vi "Gestore prove.vi"(8 "banco":i32, 9 "Status":refnum<vi>, 11 "Queue Name":string) -> ()   [LabVIEW 2019]
uses:
  TypeDef/Cluster INFO.ctl
  TypeDef/WT SELECTION.ctl
  TypeDef/Definizione linea.ctl
  TypeDef/Collegamenti_elettrici.ctl
  TypeDef/Control Calcoli.ctl
  Global prova in corso.vi
panel:
  out "Scale misura res":T1
  out "%VALVOLE":dbl[][](array[numeric])
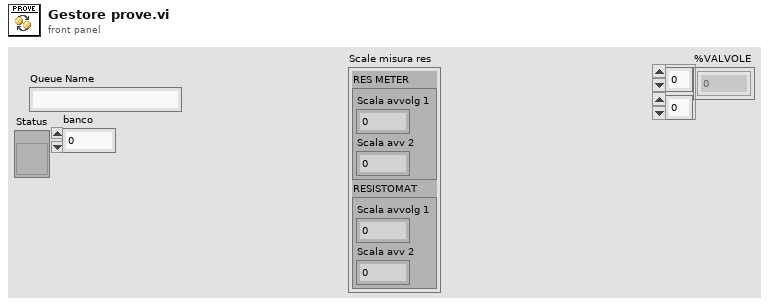
[diagram p1: front panel]
types:
  T1 = cluster{"RES METER":cluster{"Scala avvolg 1":u16, "Scala avv 2":u16}, "RESISTOMAT":cluster{"Scala avvolg 1":u16, "Scala avv 2":u16}}
  T2 = typedef "Cluster INFO.ctl" = cluster{"Scelta wattmetro":cluster{"Wattmetro":T3}, "SET RPM":dbl, "SET TEMP":dbl, "Array banchi":T4[], "Array valvole linee avvio/fermata":cluster{"Valvole avvio":cluster{"Set valvole avvio?":bool, "% valvole avvio":dbl[]}, "Valvole fermata":cluster{"Set valvole fermata?":bool, "% valvole fermata":dbl[]}}[], "banco selezionato":i8, "Nomi valvole prop sistema":string[], "canale-- sensore":string[][], "Attriti B1":dbl[][], "Attriti B2":dbl[][], "Collegamento elettrico":cluster{"ALIMENTAZIONE ELETTRICA":T5, "ID":i16, "#rami freddo\\eq term resmeter":i16, "#rami riscaldamento resmeter":i16, "#rami freddo\\eq term resistomat":i16, "#rami riscaldamento resistomat":i16, "CALCOLI":T6}, "lingua":i16, "Costanti collaudo":cluster{"P [bar]":dbl, "T amb. [°C]":dbl, "Umidità [%]":dbl, "T acqua [°C] 2":dbl}, "OPZIONI MISURE RES":cluster{"MISURA A FREDDO":enum16{"NESSUNO", "RESISTOMAT", "RES METER", "ENTRAMBI"}, "MISURA EQ. TERMICO":enum16{"NESSUNO", "RESISTOMAT", "RES METER", "ENTRAMBI"}, "MISURA DT PROVA IN CORSO":enum16{"NESSUNO", "RESISTOMAT - CON FERMATE", "RES METER - CON FERMATE", "RES METER - CONTINUO"}, "MISURE PRIMA E DOPO":enum16{"NESSUNO", "RESISTOMAT", "RES METER"}, "STRUMENTI PRESENTI":enum16{"NESSUNO", "RESISTOMAT", "RES METER", "ENTRAMBI"}}, "Dati targa motore":cluster{"Vnom":dbl, "Fnom":dbl, "Inom":dbl, "Cnom":dbl, "Npoli":dbl, "Scorta 1":dbl, "Scorta 2":dbl, "Scorta 3":dbl}}
  T3 = typedef "WT SELECTION.ctl" = enum32{"No Selection", "WT230", "WT1600", "WT1800", "WT330", "VIW", "APLUS"}
  T4 = typedef "Definizione linea.ctl" = cluster{"Nome":string, "Tors. scala1":i32, "Tors. scala2":i32, "rpm":i32, "TAMB":i32, "Indici Temperature":i16[], "Indice freno":i16, "alimentatore trifase":i16, "alimentatore monofase":i16, "alimentatore dc arm":i16, "alimentatore dc ecc":i16, "alimentatore dc mp":i16}
  T5 = typedef "Collegamenti_elettrici.ctl" = enum16{"AC TRIFASE", "AC TRIFASE + FRENO", "AC MONOFASE", "DC CON ECCITAZIONE", "DC CON ECCITAZIONE + FRENO", "DC NO ECCITAZIONE", "DC NO ECCITAZIONE + FRENO", "FRENO TRASC + AFE", "SOLO FRENO", "CARICO RESISTIVO", "GENERICO", "SOLO ACQUISITORE", "SCORTA 4", "SCORTA 5", "SCORTA 6"}
  T6 = typedef "Control Calcoli.ctl" = enum16{"AC TRIFASE", "AC MONOFASE", "DC ECCITAZIONE", "DC NO ECCITAZIONE", "POMPA TRIFASE", "POMPA MONOFASE", "GENERICO", "TRASFORMATORE", "ALTERNATORE TRASCINATO", "GRUPPO ELETTROGENO"}
  T7 = cluster{"Array of elements":cluster{"String":string, "variant":variant}[], "Single element":cluster{"String":string, "variant":variant}, "enque at\nopposite end (F)":bool, "no replications (F)":bool}
  T8 = cluster{"Prova":string, "MAN/AUTO":bool, "Tipo motore pompa":enum16{"Monofase", "Trifase"}}
  T9 = cluster{"Res Ch1":dbl, "Res Ch2":dbl, "tAMB":dbl, "Res Ch3":dbl}
  T10 = cluster{"Res Ch1":dbl, "Res Ch2":dbl, "tAMB":dbl}
  T11 = cluster{"ALIMENTAZIONE ELETTRICA":T5, "ID":i16, "#rami freddo\\eq term resmeter":i16, "#rami riscaldamento resmeter":i16, "#rami freddo\\eq term resistomat":i16, "#rami riscaldamento resistomat":i16, "CALCOLI":T6}
  T12 = cluster{"MISURA A FREDDO":enum16{"NESSUNO", "RESISTOMAT", "RES METER", "ENTRAMBI"}, "MISURA EQ. TERMICO":enum16{"NESSUNO", "RESISTOMAT", "RES METER", "ENTRAMBI"}, "MISURA DT PROVA IN CORSO":enum16{"NESSUNO", "RESISTOMAT - CON FERMATE", "RES METER - CON FERMATE", "RES METER - CONTINUO"}, "MISURE PRIMA E DOPO":enum16{"NESSUNO", "RESISTOMAT", "RES METER"}, "STRUMENTI PRESENTI":enum16{"NESSUNO", "RESISTOMAT", "RES METER", "ENTRAMBI"}}
  T13 = enum16{"NESSUNO", "RESISTOMAT", "RES METER", "ENTRAMBI"}
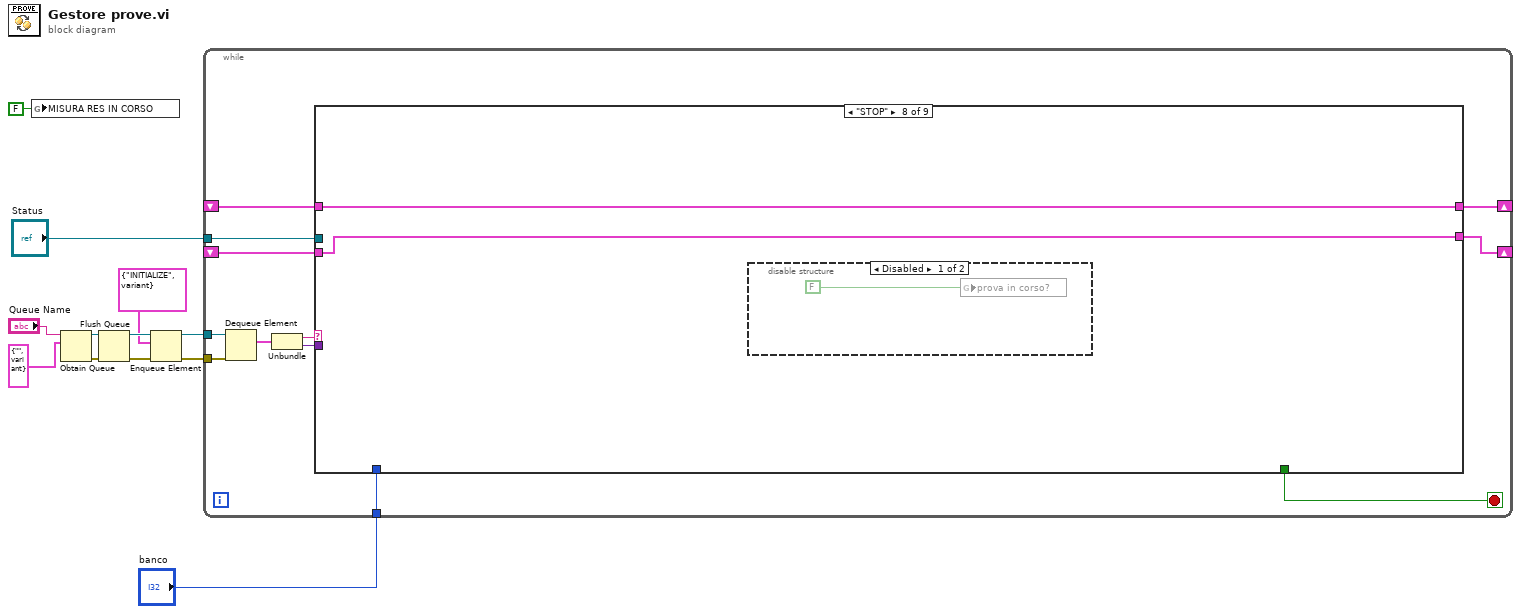
[diagram p0: block diagram]
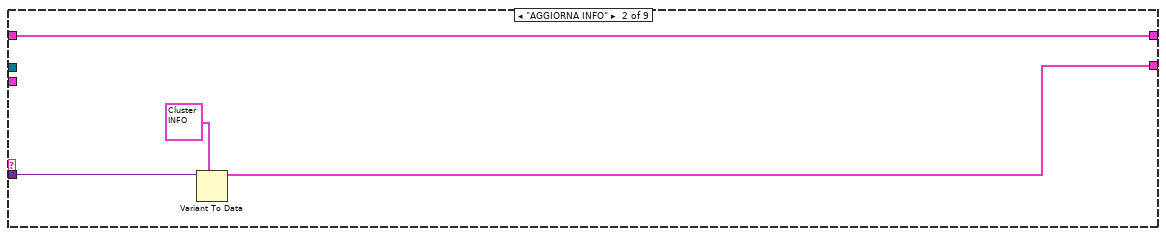
[diagram p3: hidden frame]
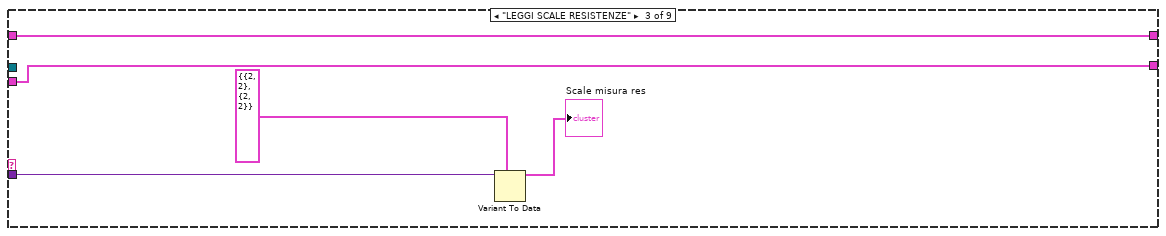
[diagram p4: hidden frame]
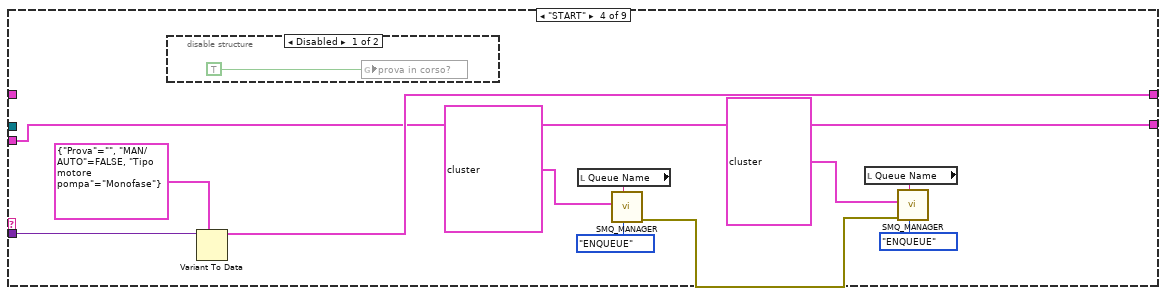
[diagram p5: hidden frame]
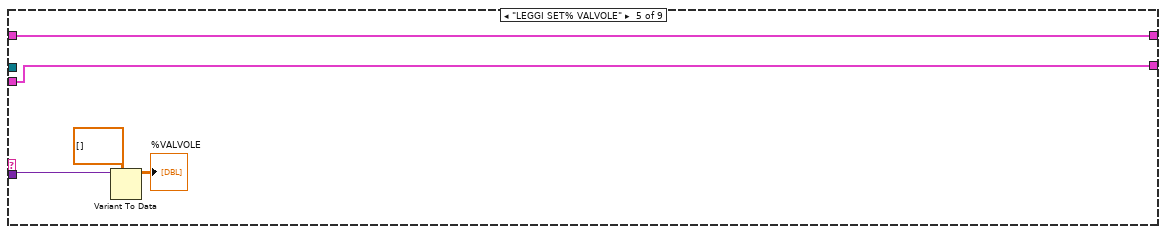
[diagram p7: hidden frame]
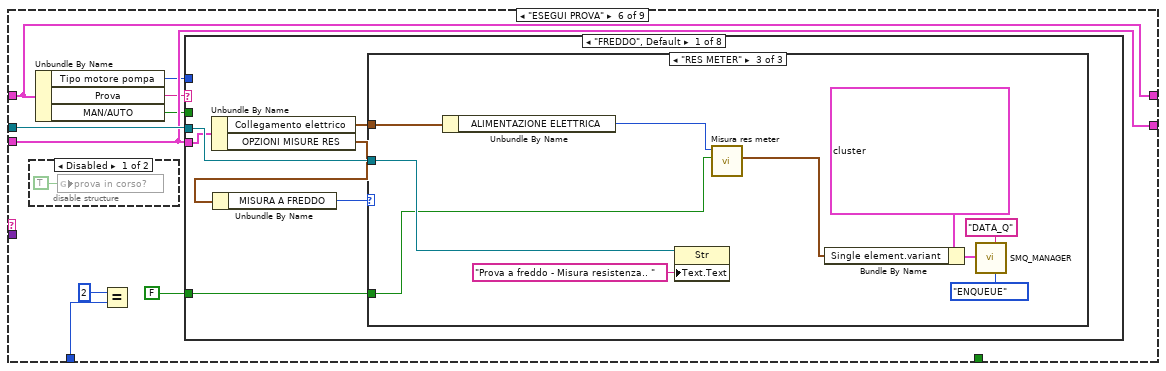
[diagram p8: hidden frame]
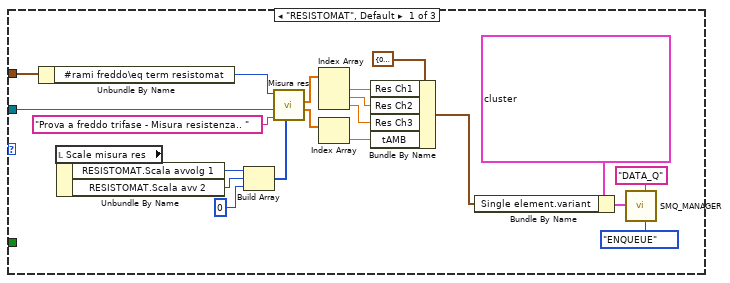
[diagram p10: hidden frame]
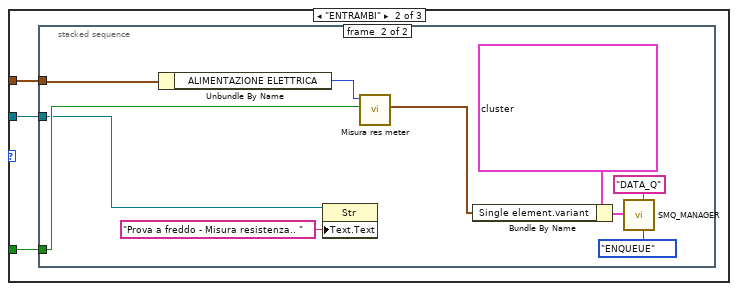
[diagram p11: hidden frame]
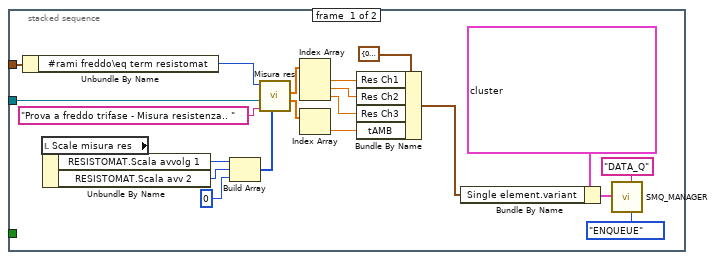
[diagram p12: hidden frame]
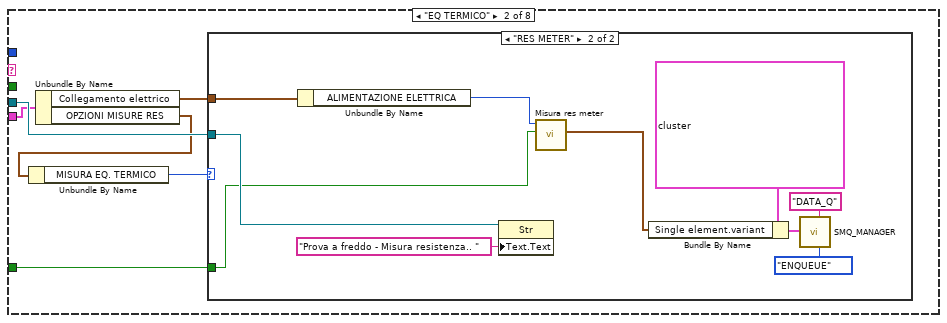
[diagram p13: hidden frame]
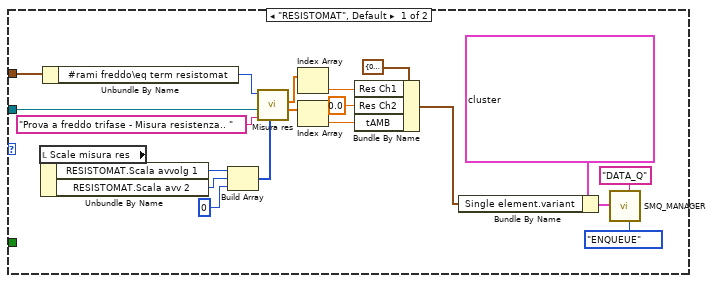
[diagram p14: hidden frame]
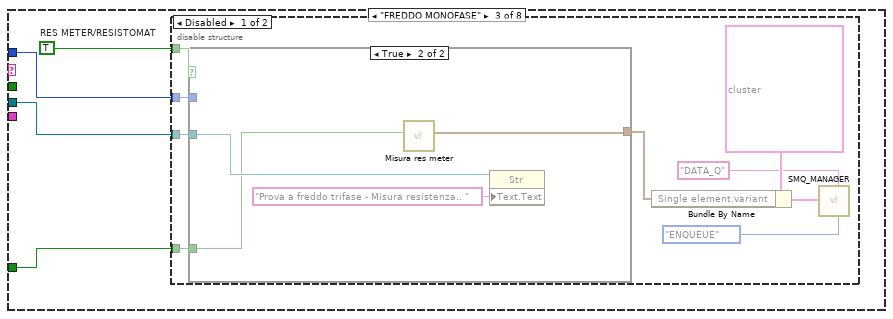
[diagram p15: hidden frame]
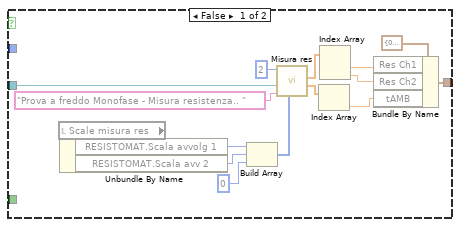
[diagram p16: hidden frame]
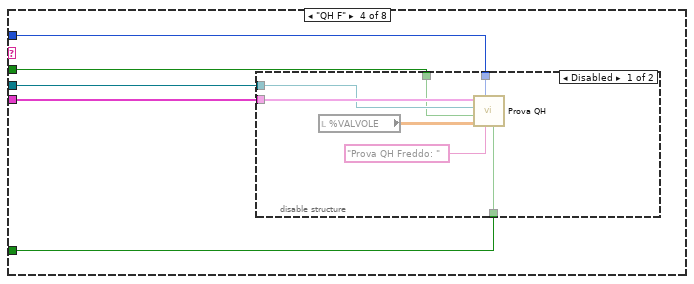
[diagram p18: hidden frame]
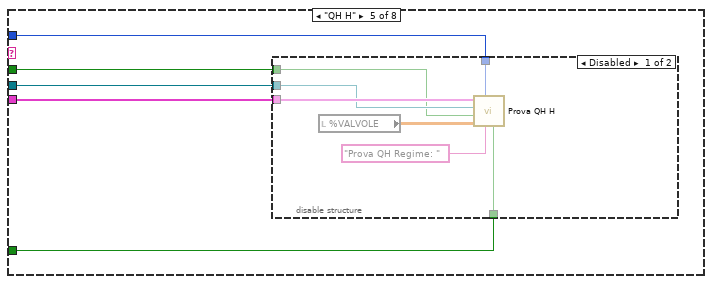
[diagram p20: hidden frame]
diagram:
  n1 = global write "Global prova in corso.vi" "MISURA RES IN CORSO"(FALSE ("prova in corso?")) -> ()
  n2 = Obtain Queue(name (unnamed)="Queue Name", element data type=cluster{"String":string, "variant":variant} {"String"="", "variant"=variant} ("element")) -> (queue out=w6:refnum<queue>, error out=w7:errorcluster)  [unwired: 3 in, 1 out]
  n3 = Flush Queue(queue=w6, error in (no error)=w7) -> (queue out=w9:refnum<queue>, error out=w10:errorcluster)  [unwired: 1 out]
  n4 = Enqueue Element(queue=w9, element=cluster{"String":string, "variant":variant} {"String"="INITIALIZE", "variant"=variant}, error in (no error)=w10) -> (queue out=w11:refnum<queue>, error out=w12:errorcluster)  [unwired: 1 in, 1 out]
  n5 = while {
    tunnel: w11 -> [w23]
    tunnel: w12 -> [w22]
    shift-right: [w19] -> _
    shift-left: _ -> [w18]
    tunnel: "Status" -> [w17]
    shift-right: [w15] -> _
    shift-left: _ -> [w14]
    tunnel: "banco" -> [w13]
    stop <- w16 stop-if-true
    n6 = Dequeue Element(queue=w23, error in (no error)=w22) -> (element=w24:cluster{"String":string, "variant":variant})  [unwired: 1 in, 3 out]
    n7 = Unbundle(w24) -> ("String"=w21:string, "variant"=w20:variant)
    n8 = case shown="\"STOP\"" w21 {
      tunnel: w20 -> [_ w30 w35 w43 w50 _ _ _ _]
      tunnel: [w26 w29 w33 w42 w52 w59 w261 w263 w266] -> w19
      tunnel: w18 -> [w26 w29 w33 _ w52 w59 w261 w263 w266]
      tunnel: w17 -> [_ _ _ _ _ w61 _ _ _]
      tunnel: [_ _ _ _ _ _ _ _ TRUE] -> w16
      tunnel: [w25 w28 w32 w41 w51 w60 w260 w262 w265] -> w15
      tunnel: w14 -> [w25 _ w32 w41 w51 w60 w260 w262 w265]
      tunnel: w13 -> [_ _ _ _ _ w55 _ _ _]
      frame "INITIALIZE", Default {
      }
      frame "AGGIORNA INFO" {
        n9 = Variant To Data(type=T2 {"Scelta wattmetro"={"Wattmetro"=enum."No Selection"}, "SET RPM"=0.0, "SET TEMP"=0.0, "Array banchi"=[{"Nome"="Elettropompa", "Tors. scala1"=0, "Tors. scala2"=0, "rpm"=0, "TAMB"=0, "Indici Temperature"=[0, 1], "Indice freno"=1, "alimentatore trifase"=0, "alimentatore monofase"=0, "alimentatore dc arm"=0, "alimentatore dc ecc"=0, "alimentatore dc mp"=0}, {"Nome"="Sommersa", "Tors. scala1"=0, "Tors. scala2"=0, "rpm"=0, "TAMB"=1, "Indici Temperature"=[0, 1], "Indice freno"=0, "alimentatore trifase"=0, "alimentatore monofase"=0, "alimentatore dc arm"=0, "alimentatore dc ecc"=0, "alimentatore dc mp"=0}], "Array valvole linee avvio/fermata"=[], "banco selezionato"=0, "Nomi valvole prop sistema"=[], "canale-- sensore"=[], "Attriti B1"=[], "Attriti B2"=[], "Collegamento elettrico"={"ALIMENTAZIONE ELETTRICA"=enum."AC TRIFASE", "ID"=0, "#rami freddo\\eq term resmeter"=0, "#rami riscaldamento resmeter"=0, "#rami freddo\\eq term resistomat"=0, "#rami riscaldamento resistomat"=0, "CALCOLI"=enum."AC TRIFASE"}, "lingua"=0, "Costanti collaudo"={"P [bar]"=0.0, "T amb. [°C]"=0.0, "Umidità [%]"=0.0, "T acqua [°C] 2"=0.0}, "OPZIONI MISURE RES"={"MISURA A FREDDO"=enum."RESISTOMAT", "MISURA EQ. TERMICO"=enum."RESISTOMAT", "MISURA DT PROVA IN CORSO"=enum."RESISTOMAT - CON FERMATE", "MISURE PRIMA E DOPO"=enum."RESISTOMAT", "STRUMENTI PRESENTI"=enum."NESSUNO"}, "Dati targa motore"={"Vnom"=0.0, "Fnom"=0.0, "Inom"=0.0, "Cnom"=0.0, "Npoli"=0.0, "Scorta 1"=0.0, "Scorta 2"=0.0, "Scorta 3"=0.0}} ("Cluster INFO"), Variant=w30) -> (data=w28:T2)  [unwired: 1 in, 1 out]
      }
      frame "LEGGI SCALE RESISTENZE" {
        n10 = Variant To Data(type=T1 {"RES METER"={"Scala avvolg 1"=2, "Scala avv 2"=2}, "RESISTOMAT"={"Scala avvolg 1"=2, "Scala avv 2"=2}} ("Scale Misura res"), Variant=w35) -> (data=→"Scale misura res":T1)  [unwired: 1 in, 1 out]
      }
      frame "START" {
        n11 = disable-structure shown="Disabled" {
          frame Disabled {
            n12 = global write "Global prova in corso.vi" "prova in corso?"(TRUE ("prova in corso?")) -> ()
          }
          frame Enabled {
          }
        }
        n13 = Variant To Data(type=T8 {"Prova"="", "MAN/AUTO"=FALSE, "Tipo motore pompa"=enum."Monofase"} ("output cluster"), Variant=w43) -> (data=w42:T8)  [unwired: 1 in, 1 out]
        n14 = local read "Queue Name"() -> (w45:string)
        n15 = call <userlib>:"SMQ_MANAGER.vi"("Function"=enum16{"INITIALIZE", "ENQUEUE", "STOP ALL"}."ENQUEUE", "Queue name"=w45, "Enqueue cluster"=T7 {"Array of elements"=[], "Single element"={"String"="ESEGUI PROVA", "variant"=variant}, "enque at\nopposite end (F)"=FALSE, "no replications (F)"=FALSE}) -> ("error out"=w36:errorcluster)  [unwired: 8 in]
        n16 = local read "Queue Name"() -> (w38:string)
        n17 = call <userlib>:"SMQ_MANAGER.vi"("Function"=enum16{"INITIALIZE", "ENQUEUE", "STOP ALL"}."ENQUEUE", "Queue name"=w38, "error in (no error)"=w36, "Enqueue cluster"=T7 {"Array of elements"=[], "Single element"={"String"="FINE PROVA", "variant"=variant}, "enque at\nopposite end (F)"=FALSE, "no replications (F)"=FALSE}) -> ()  [unwired: 7 in, 1 out]
      }
      frame "LEGGI SET% VALVOLE" {
        n18 = Variant To Data(type=dbl[][] [], Variant=w50) -> (data=→"%VALVOLE":dbl[][])  [unwired: 1 in, 1 out]
      }
      frame "ESEGUI PROVA" {
        n19 = disable-structure shown="Disabled" {
          frame Disabled {
            n20 = global write "Global prova in corso.vi" "prova in corso?"(TRUE ("prova in corso?")) -> ()
          }
          frame Enabled {
          }
        }
        n21 = Unbundle By Name(w59) -> ("Tipo motore pompa"=w57:enum16{"Monofase", "Trifase"}, "Prova"=w58:string, "MAN/AUTO"=w56:bool)
        n22 = Equal?(x=2, y=w55) -> ()  [unwired: 1 out]
        n23 = case shown="\"FREDDO\", Default" w58 {
          tunnel: w61 -> [w68 w139 w173 w205 w217 w228 w237 w251]
          tunnel: w60 -> [w66 w137 _ w206 w218 w229 w239 w253]
          tunnel: w57 -> [_ _ w170 w204 w216 w227 w238 w252]
          tunnel: w56 -> [_ _ _ w203 w215 _ _ w250]
          tunnel: FALSE -> [w67 w138 w171 w202 w214 w226 w236 _]
          frame "FREDDO", Default {
            n24 = Unbundle By Name(w66) -> ("Collegamento elettrico"=w63:T11, "OPZIONI MISURE RES"=w65:T12)
            n25 = Unbundle By Name(w65) -> ("MISURA A FREDDO"=w64:T13)
            n26 = case shown="\"RES METER\"" w64 {
              tunnel: w68 -> [w89 w92 w133]
              tunnel: w67 -> [_ w90 w131]
              tunnel: w63 -> [w74 w91 w125]
              frame "RESISTOMAT", Default {
                n27 = Unbundle By Name(w74) -> ("#rami freddo\\eq term resistomat"=w73:i16)
                n28 = local read "Scale misura res"() -> (w88:T1)
                n29 = Unbundle By Name(w88) -> ("RESISTOMAT.Scala avvolg 1"=w87:u16, "RESISTOMAT.Scala avv 2"=w86:u16)
                n30 = Build Array(w87, w86, u16 0 ("element")) -> (w85:u16[])
                n31 = call "Misura res.vi"("Scala per ramo"=w85, "String"="Prova a freddo trifase - Misura resistenza.. ", "Status"=w89, "N°rami"=w73) -> ("temperature amb"=w82:dbl[], "Valori res (ohm)"=w81:dbl[])  [unwired: 5 in, 1 out]
                n32 = Index Array(array=w81) -> (element #1=w80:dbl, element #2=w70:dbl, element #3=w69:dbl)  [unwired: 3 in]
                n33 = Index Array(array=w82) -> (element=w71:dbl)  [unwired: 1 in]
                n34 = Bundle By Name(cluster=T9 {"Res Ch1"=0.0, "Res Ch2"=0.0, "tAMB"=0.0, "Res Ch3"=0.0} ("FREDDO resistomat"), "Res Ch1"=w80, "Res Ch2"=w70, "Res Ch3"=w69, "tAMB"=w71) -> (w75:T9)
                n35 = Bundle By Name(cluster=T7 {"Array of elements"=[], "Single element"={"String"="READ RES FREDDO RESISTOMAT", "variant"=variant}, "enque at\nopposite end (F)"=FALSE, "no replications (F)"=FALSE} ("Enqueue cluster"), "Single element.variant"=w75) -> (w79:T7)
                n36 = call <userlib>:"SMQ_MANAGER.vi"("Function"=enum16{"INITIALIZE", "ENQUEUE", "STOP ALL"}."ENQUEUE", "Queue name"="DATA_Q", "Enqueue cluster"=w79) -> ()  [unwired: 8 in, 1 out]
              }
              frame "ENTRAMBI" {
                n37 = stacked-sequence {
                  tunnel: w92 -> [w113 w114]
                  tunnel: w91 -> [w98 w116]
                  tunnel: w90 -> [_ w115]
                  frame #0 {
                    n38 = Unbundle By Name(w98) -> ("#rami freddo\\eq term resistomat"=w97:i16)
                    n39 = local read "Scale misura res"() -> (w112:T1)
                    n40 = Unbundle By Name(w112) -> ("RESISTOMAT.Scala avvolg 1"=w111:u16, "RESISTOMAT.Scala avv 2"=w110:u16)
                    n41 = Build Array(w111, w110, u16 0 ("element")) -> (w109:u16[])
                    n42 = call "Misura res.vi"("Scala per ramo"=w109, "String"="Prova a freddo trifase - Misura resistenza.. ", "Status"=w113, "N°rami"=w97) -> ("temperature amb"=w106:dbl[], "Valori res (ohm)"=w105:dbl[])  [unwired: 5 in, 1 out]
                    n43 = Index Array(array=w105) -> (element #1=w104:dbl, element #2=w94:dbl, element #3=w93:dbl)  [unwired: 3 in]
                    n44 = Index Array(array=w106) -> (element=w95:dbl)  [unwired: 1 in]
                    n45 = Bundle By Name(cluster=T9 {"Res Ch1"=0.0, "Res Ch2"=0.0, "tAMB"=0.0, "Res Ch3"=0.0} ("FREDDO resistomat"), "Res Ch1"=w104, "Res Ch2"=w94, "Res Ch3"=w93, "tAMB"=w95) -> (w99:T9)
                    n46 = Bundle By Name(cluster=T7 {"Array of elements"=[], "Single element"={"String"="READ RES FREDDO RESISTOMAT", "variant"=variant}, "enque at\nopposite end (F)"=FALSE, "no replications (F)"=FALSE} ("Enqueue cluster"), "Single element.variant"=w99) -> (w103:T7)
                    n47 = call <userlib>:"SMQ_MANAGER.vi"("Function"=enum16{"INITIALIZE", "ENQUEUE", "STOP ALL"}."ENQUEUE", "Queue name"="DATA_Q", "Enqueue cluster"=w103) -> ()  [unwired: 8 in, 1 out]
                  }
                  frame #1 {
                    n48 = Unbundle By Name(w116) -> ("ALIMENTAZIONE ELETTRICA"=w117:T5)
                    n49 = property class="Str"(reference=w114, "Text.Text"="Prova a freddo - Misura resistenza.. " ("String")) -> ()  [unwired: 1 in, 2 out]
                    n50 = call "Misura res meter.vi"("solo lettura?"=w115, "ALIMENTAZIONE ELETTRICA"=w117) -> ("FREDDO"=w118:T9)  [unwired: 9 in]
                    n51 = Bundle By Name(cluster=T7 {"Array of elements"=[], "Single element"={"String"="READ RES FREDDO RES METER", "variant"=variant}, "enque at\nopposite end (F)"=FALSE, "no replications (F)"=FALSE} ("Enqueue cluster"), "Single element.variant"=w118) -> (w122:T7)
                    n52 = call <userlib>:"SMQ_MANAGER.vi"("Function"=enum16{"INITIALIZE", "ENQUEUE", "STOP ALL"}."ENQUEUE", "Queue name"="DATA_Q", "Enqueue cluster"=w122) -> ()  [unwired: 8 in, 1 out]
                  }
                }
              }
              frame "RES METER" {
                n53 = Unbundle By Name(w125) -> ("ALIMENTAZIONE ELETTRICA"=w124:T5)
                n54 = property class="Str"(reference=w133, "Text.Text"="Prova a freddo - Misura resistenza.. " ("String")) -> ()  [unwired: 1 in, 2 out]
                n55 = call "Misura res meter.vi"("solo lettura?"=w131, "ALIMENTAZIONE ELETTRICA"=w124) -> ("FREDDO"=w126:T9)  [unwired: 9 in]
                n56 = Bundle By Name(cluster=T7 {"Array of elements"=[], "Single element"={"String"="READ RES FREDDO RES METER", "variant"=variant}, "enque at\nopposite end (F)"=FALSE, "no replications (F)"=FALSE} ("Enqueue cluster"), "Single element.variant"=w126) -> (w130:T7)
                n57 = call <userlib>:"SMQ_MANAGER.vi"("Function"=enum16{"INITIALIZE", "ENQUEUE", "STOP ALL"}."ENQUEUE", "Queue name"="DATA_Q", "Enqueue cluster"=w130) -> ()  [unwired: 8 in, 1 out]
              }
            }
          }
          frame "EQ TERMICO" {
            n58 = Unbundle By Name(w137) -> ("Collegamento elettrico"=w134:T11, "OPZIONI MISURE RES"=w136:T12)
            n59 = Unbundle By Name(w136) -> ("MISURA EQ. TERMICO"=w135:T13)
            n60 = case shown="\"RES METER\"" w135 {
              tunnel: w139 -> [w159 w169]
              tunnel: w138 -> [_ w167]
              tunnel: w134 -> [w141 w161]
              frame "RESISTOMAT", Default {
                n61 = local read "Scale misura res"() -> (w158:T1)
                n62 = Unbundle By Name(w158) -> ("RESISTOMAT.Scala avvolg 1"=w157:u16, "RESISTOMAT.Scala avv 2"=w156:u16)
                n63 = Unbundle By Name(w141) -> ("#rami freddo\\eq term resistomat"=w140:i16)
                n64 = Build Array(w157, w156, u16 0 ("element")) -> (w155:u16[])
                n65 = call "Misura res.vi"("Scala per ramo"=w155, "String"="Prova a freddo trifase - Misura resistenza.. ", "Status"=w159, "N°rami"=w140) -> ("temperature amb"=w152:dbl[], "Valori res (ohm)"=w148:dbl[])  [unwired: 5 in, 1 out]
                n66 = Index Array(array=w148) -> (element=w147:dbl)  [unwired: 1 in]
                n67 = Index Array(array=w152) -> (element=w150:dbl)  [unwired: 1 in]
                n68 = Bundle By Name(cluster=T10 {"Res Ch1"=0.0, "Res Ch2"=0.0, "tAMB"=0.0} ("Cluster FREDDO"), "Res Ch1"=w147, "Res Ch2"=0.0, "tAMB"=w150) -> (w142:T10)
                n69 = Bundle By Name(cluster=T7 {"Array of elements"=[], "Single element"={"String"="READ RES FREDDO RESISTOMAT", "variant"=variant}, "enque at\nopposite end (F)"=FALSE, "no replications (F)"=FALSE} ("Enqueue cluster"), "Single element.variant"=w142) -> (w146:T7)
                n70 = call <userlib>:"SMQ_MANAGER.vi"("Function"=enum16{"INITIALIZE", "ENQUEUE", "STOP ALL"}."ENQUEUE", "Queue name"="DATA_Q", "Enqueue cluster"=w146) -> ()  [unwired: 8 in, 1 out]
              }
              frame "RES METER" {
                n71 = Unbundle By Name(w161) -> ("ALIMENTAZIONE ELETTRICA"=w160:T5)
                n72 = property class="Str"(reference=w169, "Text.Text"="Prova a freddo - Misura resistenza.. " ("String")) -> ()  [unwired: 1 in, 2 out]
                n73 = call "Misura res meter.vi"("solo lettura?"=w167, "ALIMENTAZIONE ELETTRICA"=w160) -> ("FREDDO"=w162:T9)  [unwired: 9 in]
                n74 = Bundle By Name(cluster=T7 {"Array of elements"=[], "Single element"={"String"="READ RES FREDDO RESISTOMAT", "variant"=variant}, "enque at\nopposite end (F)"=FALSE, "no replications (F)"=FALSE} ("Enqueue cluster"), "Single element.variant"=w162) -> (w166:T7)
                n75 = call <userlib>:"SMQ_MANAGER.vi"("Function"=enum16{"INITIALIZE", "ENQUEUE", "STOP ALL"}."ENQUEUE", "Queue name"="DATA_Q", "Enqueue cluster"=w166) -> ()  [unwired: 8 in, 1 out]
              }
            }
          }
          frame "FREDDO MONOFASE" {
            w172 = TRUE  # RES METER/RESISTOMAT
            n76 = disable-structure shown="Disabled" {
              disable-tunnel: w173 -> [w182 _]
              disable-tunnel: w172 -> [w176 _]
              disable-tunnel: w171 -> [w175 _]
              disable-tunnel: w170 -> [w174 _]
              frame Disabled {
                n77 = case shown="True" w176 {
                  tunnel: w182 -> [w197 w200]
                  tunnel: [w186 w201] -> w177
                  tunnel: w175 -> [_ w198]
                  tunnel: w174 -> [_ _]
                  frame False {
                    n78 = local read "Scale misura res"() -> (w196:T1)
                    n79 = Unbundle By Name(w196) -> ("RESISTOMAT.Scala avvolg 1"=w195:u16, "RESISTOMAT.Scala avv 2"=w194:u16)
                    n80 = Build Array(w195, w194, u16 0 ("element")) -> (w193:u16[])
                    n81 = call "Misura res.vi"("Scala per ramo"=w193, "String"="Prova a freddo Monofase - Misura resistenza.. ", "Status"=w197, "N°rami"=2) -> ("temperature amb"=w189:dbl[], "Valori res (ohm)"=w185:dbl[])  [unwired: 5 in, 1 out]
                    n82 = Index Array(array=w189) -> (element=w187:dbl)  [unwired: 1 in]
                    n83 = Index Array(array=w185) -> (element #1=w184:dbl, element #2=w183:dbl)  [unwired: 2 in]
                    n84 = Bundle By Name(cluster=T10 {"Res Ch1"=0.0, "Res Ch2"=0.0, "tAMB"=0.0} ("Cluster FREDDO"), "Res Ch1"=w184, "Res Ch2"=w183, "tAMB"=w187) -> (w186:T10)
                  }
                  frame True {
                    n85 = call "Misura res meter.vi"("solo lettura?"=w198) -> ("FREDDO"=w201:T9)  [unwired: 10 in]
                    n86 = property class="Str"(reference=w200, "Text.Text"="Prova a freddo trifase - Misura resistenza.. " ("String")) -> ()  [unwired: 1 in, 2 out]
                  }
                }
                n87 = Bundle By Name(cluster=T7 {"Array of elements"=[], "Single element"={"String"="READ RES FREDDO", "variant"=variant}, "enque at\nopposite end (F)"=FALSE, "no replications (F)"=FALSE} ("Enqueue cluster"), "Single element.variant"=w177) -> (w181:T7)
                n88 = call <userlib>:"SMQ_MANAGER.vi"("Function"=enum16{"INITIALIZE", "ENQUEUE", "STOP ALL"}."ENQUEUE", "Queue name"="DATA_Q", "Enqueue cluster"=w181) -> ()  [unwired: 8 in, 1 out]
              }
              frame Enabled {
              }
            }
          }
          frame "QH F" {
            n89 = disable-structure shown="Disabled" {
              disable-tunnel: w206 -> [w213 _]
              disable-tunnel: w205 -> [w212 _]
              disable-tunnel: w204 -> [w211 _]
              disable-tunnel: w203 -> [w210 _]
              disable-tunnel: w202 -> [w207 _]
              frame Disabled {
                n90 = local read "%VALVOLE"() -> (w209:dbl[][])
                n91 = call "Prova QH.vi"("solo acquisizione!!"=w207, "Text.Text"="Prova QH Freddo: ", "Tipo motore pompa"=w211, "Array % valvole"=w209, "Manuale F\\auto T"=w210, "Status"=w212, "input cluster"=w213) -> ()  [unwired: 5 in]
              }
              frame Enabled {
              }
            }
          }
          frame "QH H" {
            n92 = disable-structure shown="Disabled" {
              disable-tunnel: w218 -> [w225 _]
              disable-tunnel: w217 -> [w224 _]
              disable-tunnel: w216 -> [w223 _]
              disable-tunnel: w215 -> [w222 _]
              disable-tunnel: w214 -> [w219 _]
              frame Disabled {
                n93 = local read "%VALVOLE"() -> (w221:dbl[][])
                n94 = call "Prova QH H.vi"("solo acquisizione!!"=w219, "Text.Text"="Prova QH Regime: ", "Tipo motore pompa"=w223, "Array % valvole"=w221, "Manuale F\\auto T"=w222, "Status"=w224, "input cluster"=w225) -> ()  [unwired: 5 in]
              }
              frame Enabled {
              }
            }
          }
          frame "NPSH" {
            n95 = disable-structure shown="Disabled" {
              disable-tunnel: w229 -> [w235 _]
              disable-tunnel: w228 -> [w234 _]
              disable-tunnel: w227 -> [w233 _]
              disable-tunnel: w226 -> [w230 _]
              frame Disabled {
                n96 = call "Prova QH.vi"("solo acquisizione!!"=w230, "Text.Text"="Prova NPSH: ", "Tipo motore pompa"=w233, "Manuale F\\auto T"=FALSE ("Manuale F\\auto T"), "Status"=w234, "input cluster"=w235) -> ()  [unwired: 6 in]
              }
              frame Enabled {
              }
            }
          }
          frame "TERMICA" {
            n97 = disable-structure shown="Disabled" {
              disable-tunnel: w239 -> [w249 _]
              disable-tunnel: w238 -> [w247 _]
              disable-tunnel: w237 -> [w246 _]
              disable-tunnel: w236 -> [w240 _]
              frame Disabled {
                n98 = local read "Scale misura res"() -> (w245:T1)
                n99 = Unbundle By Name(w245) -> ("RESISTOMAT.Scala avvolg 1"=w244:u16, "RESISTOMAT.Scala avv 2"=w243:u16)
                n100 = Build Array(w244, w243, u16 0 ("element")) -> (w241:u16[])
                n101 = call "Prova Termica.vi"("scale res"=w241, "Tipo motore pompa"=w247, "Solo acquisizione?"=w240, "Manuale F\\auto T"=TRUE ("Manuale F\\auto T"), "Status"=w246, "input cluster"=w249) -> ()  [unwired: 6 in]
              }
              frame Enabled {
              }
            }
          }
          frame "PROCEDURA TORSIOMETRO" {
            n102 = disable-structure shown="Disabled" {
              disable-tunnel: w253 -> [w258 _]
              disable-tunnel: w252 -> [w257 _]
              disable-tunnel: w251 -> [w256 _]
              disable-tunnel: w250 -> [w255 _]
              frame Disabled {
                n103 = call "PROCEDURA TORSIOMETRO.vi"("Text.Text"="Procedura torsiometro", "Tipo motore pompa"=w257, "Manuale F\\auto T"=w255, "Status"=w256, "input cluster"=w258) -> ()  [unwired: 7 in]
              }
              frame Enabled {
              }
            }
          }
        }
      }
      frame "FINE PROVA" {
        n104 = global write "Global prova in corso.vi" "MISURA RES IN CORSO"(FALSE ("prova in corso?")) -> ()
      }
      frame "STOP" {
        n105 = disable-structure shown="Disabled" {
          frame Disabled {
            n106 = global write "Global prova in corso.vi" "prova in corso?"(FALSE ("prova in corso?")) -> ()
          }
          frame Enabled {
          }
        }
      }
      frame "EXIT" {
      }
    }
  }
